vi "Write Command Status.vi"(8 "error in (no error)":errorcluster, 10 "Command Status":T1, 11 "Command in":refnum<class "Command.lvclass">) -> (0 "error out":errorcluster, 3 "Command out":refnum<class "Command.lvclass">)   [LabVIEW 2014, in "Robot Actors.lvlib" / "Command.lvlib" / "Command.lvclass"]
uses:
  Command.lvclass
  Command Status.ctl
  Command States.ctl
  <vilib>/ActorFramework/Actor/Actor.lvclass/Actor.ctl
  Command.lvclass/Command.ctl
  Command Processor/Command Processor Messages/Updated Command Status Msg/Updated Command Status Msg.lvclass/Updated Command Status Msg.ctl
  <vilib>/ActorFramework/Message Enqueuer/Message Enqueuer.lvclass/Message Enqueuer.ctl
  <vilib>/ActorFramework/Message Enqueuer/Enqueue.vi
  <vilib>/ActorFramework/Message Priority Queue/Priority Enqueue.vi
  Command Processor/Command Processor Messages/Updated Command Status Msg/Updated Command Status Msg.lvclass
  <vilib>/ActorFramework/Actor/Actor.lvclass
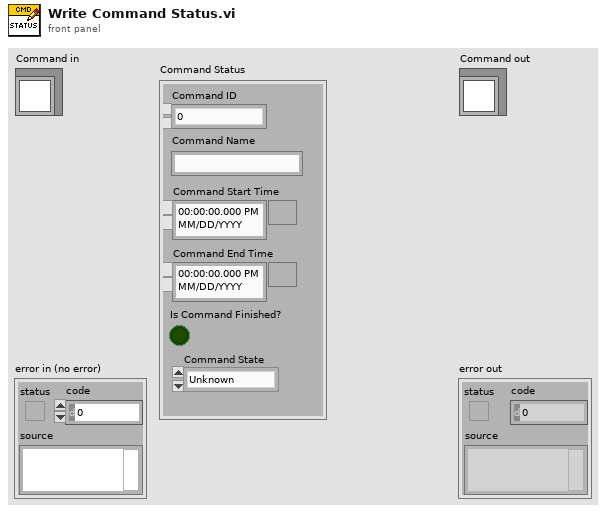
[diagram p1: front panel]
types:
  T1 = typedef "Robot Actors.lvlib/Command.lvlib/Command.lvclass/Command Status.ctl" = cluster{"Command Name":string, "Command Start Time":timestamp, "Command End Time":timestamp, "Is Command Finished?":bool, "Command ID":dbl, "Command State":T2}
  T2 = typedef "Robot Actors.lvlib/Command.lvlib/Command.lvclass/Command States.ctl" = enum16{"Unknown", "Started", "Stopped", "Finished"}
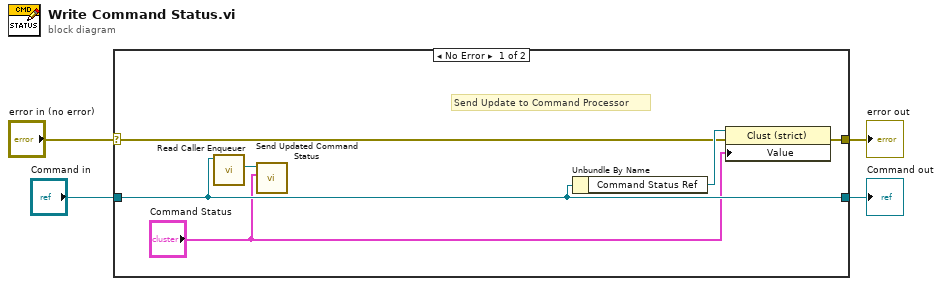
[diagram p0: block diagram]
diagram:
  n1 = case shown="No Error" "error in (no error)" {
    selector: "error in (no error)" -> [w9 w12]
    tunnel: [w8 w12] -> w3
    tunnel: [w7 w11] -> w1
    tunnel: "Command in" -> [w7 w11]
    frame No Error {
      # "Send Update to Command Processor"
      n2 = call <vilib>:"Read Caller Enqueuer.vi"("Actor"=w7) -> ("Caller Enqueuer"=w6:refnum<class "Message Enqueuer.lvclass">)  [unwired: 10 in]
      n3 = call "Send Updated Command Status.vi"("Command Status"="Command Status", "Message Enqueuer"=w6) -> ()  [unwired: 8 in, 2 out]
      n4 = Unbundle By Name(w7) -> ("Command Status Ref"=w10:refnum<vi>)
      n5 = property class="Clust (strict)"(reference=w10, error in=w9, "Value"="Command Status") -> (error out=w8:errorcluster)  [unwired: 1 out]
    }
    frame Error {
    }
  }
  "error out" <- w3
  "Command out" <- w1
